vi "Configure Serial Bus (CXPI - Trigger - Data).vi"(0 "VISA resource name":refnum<visa-resource-name>, 1 "Start Byte (0)":i32, 2 "Count Value (XX)":string="XX", 5 "Serial Bus Name (1: Serial Bus 1)":i32(ring)=1 items=["Serial Bus 1"=1, "Serial Bus 2"=2], 7 "Trigger Data (XXXXXXXXXXXX)":string="XXXXXXXXXXXX", 9 "Trigger Data Length (12)":i32=12, 11 "error in (no error)":errorcluster, 12 "Network Management Value (XX)":string="XX", 13 "Data Length Code (-1)":i32=-1) -> (4 "VISA resource name out":refnum<visa-resource-name>, 15 "error out":errorcluster)   [LabVIEW 2015, in "Agilent 2000 3000 X-Series.lvlib"]
doc: "Configures the trigger data setting of CXPI bus.\n\n<b>Note:</b>\nThis VI is only applicable for 3000T, 3000G, 4000, 6000 X-Series."
uses:
  Agilent 2000 3000 X-Series.lvlib
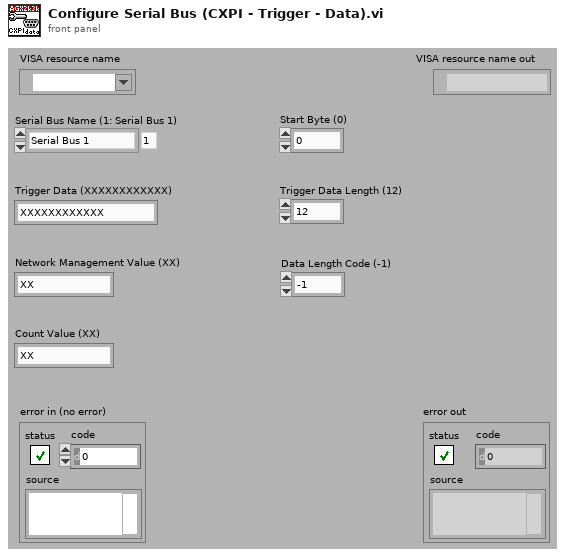
[diagram p1: front panel]
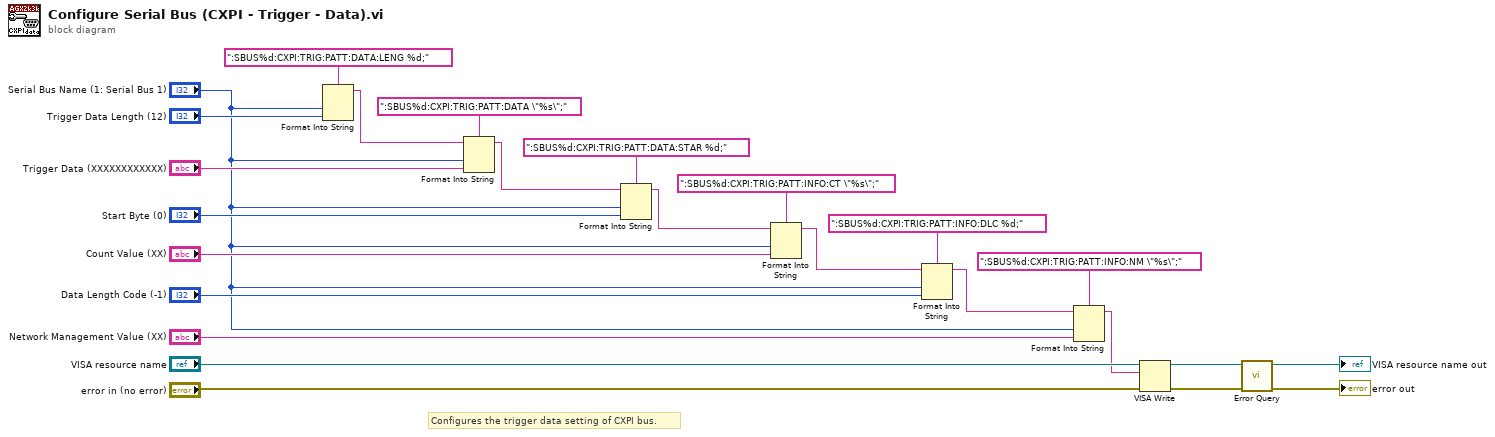
[diagram p0: block diagram]
diagram:
  # "Configures the trigger data setting of CXPI bus."
  n1 = Format Into String(format string=":SBUS%d:CXPI:TRIG:PATT:DATA:LENG %d;", "Serial Bus Name (1: Serial Bus 1)", "Trigger Data Length (12)") -> (resulting string=w23:string)  [unwired: 2 in, 1 out]
  n2 = Format Into String(format string=":SBUS%d:CXPI:TRIG:PATT:DATA \"%s\";", initial string=w23, "Serial Bus Name (1: Serial Bus 1)", "Trigger Data (XXXXXXXXXXXX)") -> (resulting string=w20:string)  [unwired: 1 in, 1 out]
  n3 = Format Into String(format string=":SBUS%d:CXPI:TRIG:PATT:DATA:STAR %d;", initial string=w20, "Serial Bus Name (1: Serial Bus 1)", "Start Byte (0)") -> (resulting string=w3:string)  [unwired: 1 in, 1 out]
  n4 = Format Into String(format string=":SBUS%d:CXPI:TRIG:PATT:INFO:CT \"%s\";", initial string=w3, "Serial Bus Name (1: Serial Bus 1)", "Count Value (XX)") -> (resulting string=w10:string)  [unwired: 1 in, 1 out]
  n5 = Format Into String(format string=":SBUS%d:CXPI:TRIG:PATT:INFO:DLC %d;", initial string=w10, "Serial Bus Name (1: Serial Bus 1)", "Data Length Code (-1)") -> (resulting string=w8:string)  [unwired: 1 in, 1 out]
  n6 = Format Into String(format string=":SBUS%d:CXPI:TRIG:PATT:INFO:NM \"%s\";", initial string=w8, "Serial Bus Name (1: Serial Bus 1)", "Network Management Value (XX)") -> (resulting string=w1:string)  [unwired: 1 in, 1 out]
  n7 = VISA Write(VISA resource name="VISA resource name", write buffer=w1, error in (no error)="error in (no error)") -> (VISA resource name out=w15:refnum<visa-resource-name>, error out=w14:errorcluster)  [unwired: 1 out]
  n8 = call "Error Query.vi"("error in (no error)"=w14, "VISA resource name"=w15) -> ("error out"=→"error out":errorcluster, "VISA resource name out"=→"VISA resource name out":refnum<visa-resource-name>)  [unwired: 6 in, 2 out]
